vi "Quick Format Core.vi"(6 "Format String":string, 8 "error in":errorcluster, 11 "GObjects":refnum<vi>[](array[refnum])) -> (2 "Successful":bool)   [LabVIEW 2019, in "Quick Format QD.lvlib"]
doc: "Recursive VI for setting the format of all selected digital, timestamp, and string controls and constants. This VI is recursive to handle elements inside of arrays and constants."
uses:
  Quick Format QD.lvlib
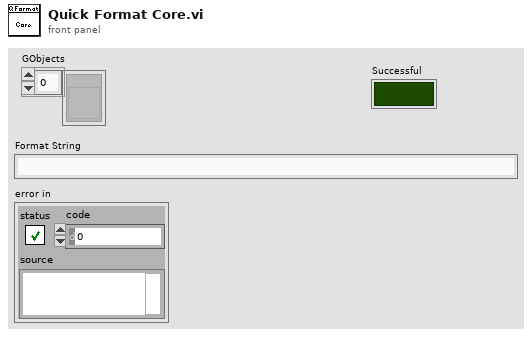
[diagram p1: front panel]
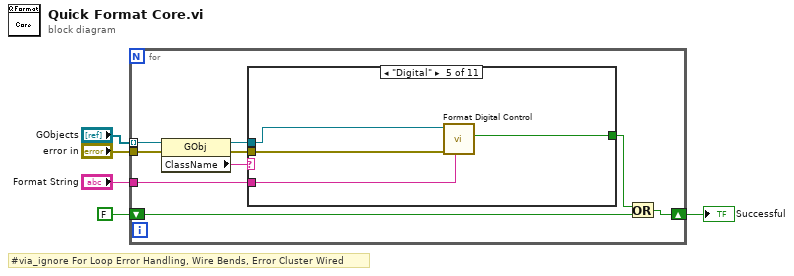
[diagram p0: block diagram]
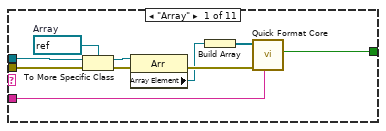
[diagram p2: hidden frame]
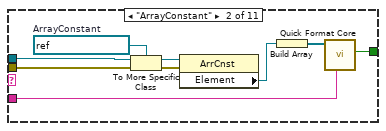
[diagram p3: hidden frame]
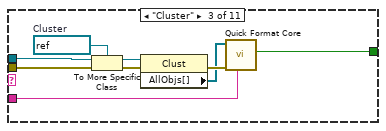
[diagram p4: hidden frame]
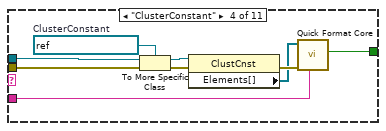
[diagram p5: hidden frame]
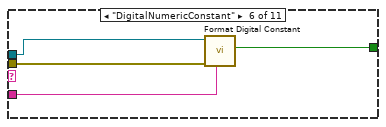
[diagram p6: hidden frame]
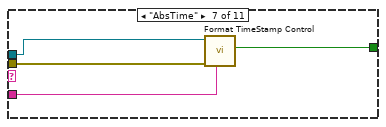
[diagram p7: hidden frame]
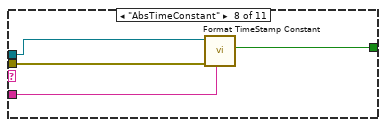
[diagram p8: hidden frame]
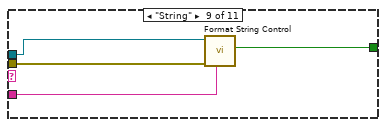
[diagram p9: hidden frame]
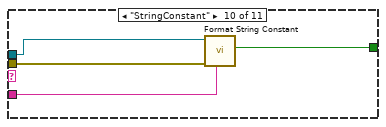
[diagram p10: hidden frame]
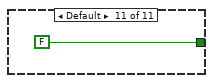
[diagram p11: hidden frame]
diagram:
  # "#via_ignore For Loop Error Handling, Wire Bends, Error Cluster Wired"
  n1 = for {
    shift-right: [w11] -> w2
    shift-left: FALSE -> [w12]
    tunnel: "GObjects" -> [w10] mode=indexing
    tunnel: "Format String" -> [w8]
    tunnel: "error in" -> [w14]
    n2 = property class="GObj"(reference=w10, error in=w14) -> (reference out=w9:refnum<vi>, error out=w13:errorcluster, "ClassName"=w6:string)
    n3 = case shown="\"Digital\"" w6 {
      tunnel: w13 -> [w24 w33 w41 w50 w55 w59 w63 w67 w71 w75 _]
      tunnel: w9 -> [w20 w30 w38 w47 w54 w58 w62 w66 w70 w74 _]
      tunnel: w8 -> [w17 w25 w34 w43 w53 w57 w61 w65 w69 w73 _]
      tunnel: [w15 w28 w35 w44 w52 w56 w60 w64 w68 w72 FALSE] -> w7
      frame "Array" {
        w21 = refnum<vi> refnum  # Array
        n4 = To More Specific Class(target class=w21, reference=w20, error in=w24) -> (specific class reference=w19:refnum<vi>, error out=w23:errorcluster)
        n5 = property class="Arr"(reference=w19, error in=w23) -> (error out=w22:errorcluster, "Array Element"=w18:refnum<vi>)  [unwired: 1 out]
        n6 = Build Array(w18) -> (w16:refnum<vi>[])
        n7 = call "Quick Format Core.vi"("Format String"=w17, "error in"=w22, "GObjects"=w16) -> ("Successful"=w15:bool)  [unwired: 8 in]
      }
      frame "ArrayConstant" {
        w31 = refnum<vi> refnum  # ArrayConstant
        n8 = To More Specific Class(target class=w31, reference=w30, error in=w33) -> (specific class reference=w29:refnum<vi>, error out=w32:errorcluster)
        n9 = property class="ArrCnst"(reference=w29, error in=w32) -> ("Element"=w27:refnum<vi>)  [unwired: 2 out]
        n10 = Build Array(w27) -> (w26:refnum<vi>[])
        n11 = call "Quick Format Core.vi"("Format String"=w25, "GObjects"=w26) -> ("Successful"=w28:bool)  [unwired: 9 in]
      }
      frame "Cluster" {
        w39 = refnum<vi> refnum  # Cluster
        n12 = To More Specific Class(target class=w39, reference=w38, error in=w41) -> (specific class reference=w37:refnum<vi>, error out=w42:errorcluster)
        n13 = property class="Clust"(reference=w37, error in=w42) -> (error out=w40:errorcluster, "AllObjs[]"=w36:refnum<vi>[])  [unwired: 1 out]
        n14 = call "Quick Format Core.vi"("Format String"=w34, "error in"=w40, "GObjects"=w36) -> ("Successful"=w35:bool)  [unwired: 8 in]
      }
      frame "ClusterConstant" {
        w48 = refnum<vi> refnum  # ClusterConstant
        n15 = To More Specific Class(target class=w48, reference=w47, error in=w50) -> (specific class reference=w46:refnum<vi>, error out=w51:errorcluster)
        n16 = property class="ClustCnst"(reference=w46, error in=w51) -> (error out=w49:errorcluster, "Elements[]"=w45:refnum<vi>[])  [unwired: 1 out]
        n17 = call "Quick Format Core.vi"("Format String"=w43, "error in"=w49, "GObjects"=w45) -> ("Successful"=w44:bool)  [unwired: 8 in]
      }
      frame "Digital" {
        n18 = call "Format Digital Control.vi"("Format String"=w53, "error in"=w55, "GObject in"=w54) -> ("Successful"=w52:bool)  [unwired: 7 in, 1 out]
      }
      frame "DigitalNumericConstant" {
        n19 = call "Format Digital Constant.vi"("Format String"=w57, "error in"=w59, "GObject in"=w58) -> ("Successful"=w56:bool)  [unwired: 7 in, 1 out]
      }
      frame "AbsTime" {
        n20 = call "Format TimeStamp Control.vi"("Format String"=w61, "error in"=w63, "GObject in"=w62) -> ("Successful"=w60:bool)  [unwired: 7 in, 1 out]
      }
      frame "AbsTimeConstant" {
        n21 = call "Format TimeStamp Constant.vi"("Format String"=w65, "error in"=w67, "GObject in"=w66) -> ("Successful"=w64:bool)  [unwired: 7 in, 1 out]
      }
      frame "String" {
        n22 = call "Format String Control.vi"("Format String"=w69, "error in"=w71, "GObject in"=w70) -> ("Successful"=w68:bool)  [unwired: 7 in, 1 out]
      }
      frame "StringConstant" {
        n23 = call "Format String Constant.vi"("Format String"=w73, "error in"=w75, "GObject in"=w74) -> ("Successful"=w72:bool)  [unwired: 7 in, 1 out]
      }
      frame Default {
      }
    }
    n24 = Or(x=w7, y=w12) -> (x .or. y?=w11:bool)
  }
  "Successful" <- w2
